vi "DataDir.vi"(1 "name":string) -> (0 "path":path)   [LabVIEW 2014]
panel:
  in  "basedir":path=path "G:/Data"
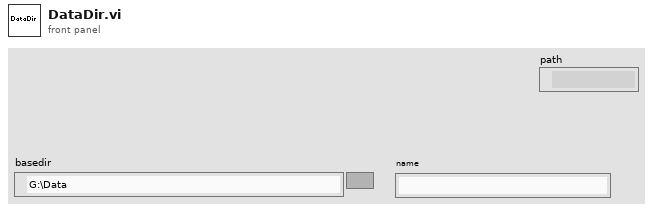
[diagram p1: front panel]
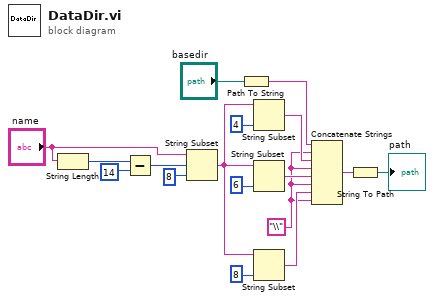
[diagram p0: block diagram]
diagram:
  w8 = "\\" ("string")
  n1 = String Length(string="name") -> (length=w17:i32)
  n2 = Subtract(x=w17, y=14) -> (x-y=w15:i32)
  n3 = String Subset(string="name", offset (0)=w15, length (rest)=8 ("length (rest)")) -> (substring=w14:string)
  n4 = Path To String(path="basedir") -> (string=w12:string)
  n5 = String Subset(string=w14, length (rest)=4 ("offset (0)")) -> (substring=w11:string)  [unwired: 1 in]
  n6 = String Subset(string=w14, length (rest)=6 ("offset (0)")) -> (substring=w10:string)  [unwired: 1 in]
  n7 = String Subset(string=w14, length (rest)=8 ("offset (0)")) -> (substring=w9:string)  [unwired: 1 in]
  n8 = Concatenate Strings(w12, w8, w11, w8, w10, w8, w9, w8) -> (w2:string)
  n9 = String To Path(string=w2) -> (path=→"path":path)
